vi "Treat Command.vi"(8 "error in (no error)":errorcluster, 11 "Channel in":refnum<class "Channel.lvclass">) -> (0 "error out":errorcluster, 3 "Channel out":refnum<class "Channel.lvclass">)   [LabVIEW 2018, in "Channel.lvclass"]
doc: "Treat the commando received from the control interface."
uses:
  Channel.lvclass
  Channel.lvclass/Channel.ctl
  State Machine/CCS_State Machine.lvclass
  Simulated_CCD_Camera/Simulated Camera.lvclass
  RxTx/CCS_RxTx.lvclass
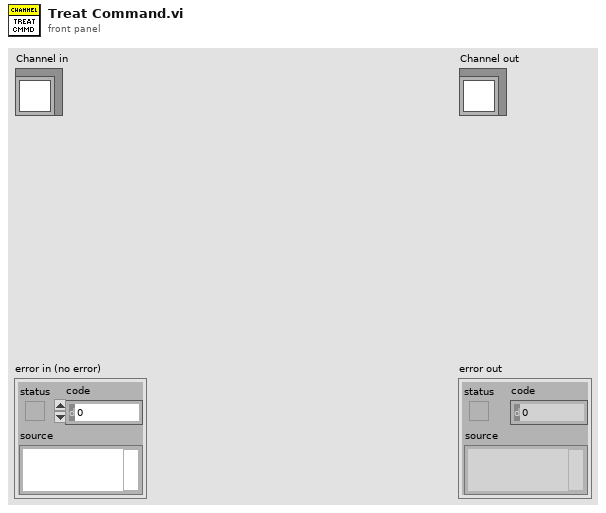
[diagram p1: front panel]
types:
  T1 = cluster{"CYCLES_DONE":u16, "LAST_IMAGE_NAME":string, "USED_DISK_SPACE":u16, "FRAMES_DONE":u16, "CCD_STATUS":string, "CURRENT_TEMPERATURE":i16, "TEMPERATURE_STATUS":string, "FRAME_EXPOSURE_TIME":sgl, "ERROR":bool, "SERIAL_NUMBER":u16, "ACQUIRING":bool, "IMAGE_INDEX":u32, "SEQS_DONE":u16}
  T2 = cluster{"COOLER_POWER_STATUS":u16, "TEMP":i32, "EXPTIME":dbl, "#FRAMES":u32, "#CYCLES":u32, "#SEQS":u32, "WAVEPLATE_POS":u16}
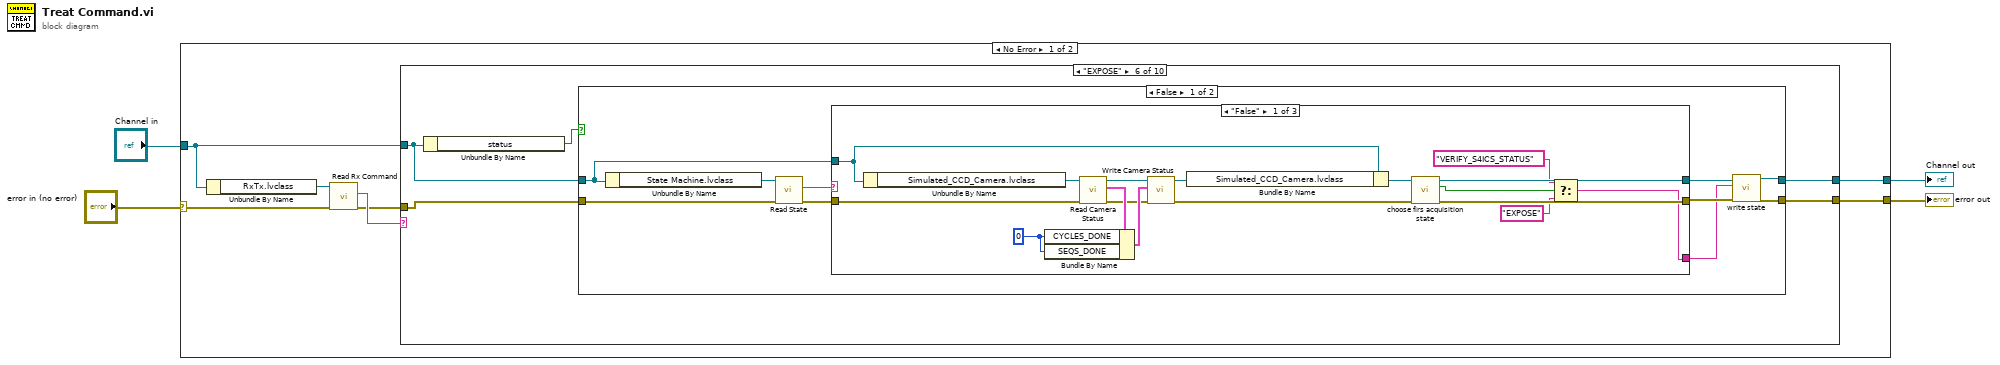
[diagram p0: block diagram]
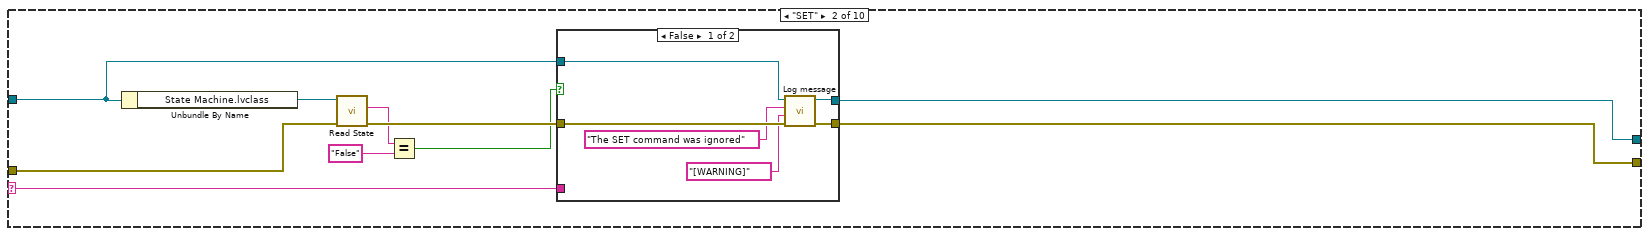
[diagram p3: hidden frame]
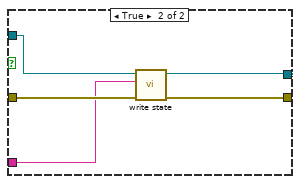
[diagram p4: hidden frame]
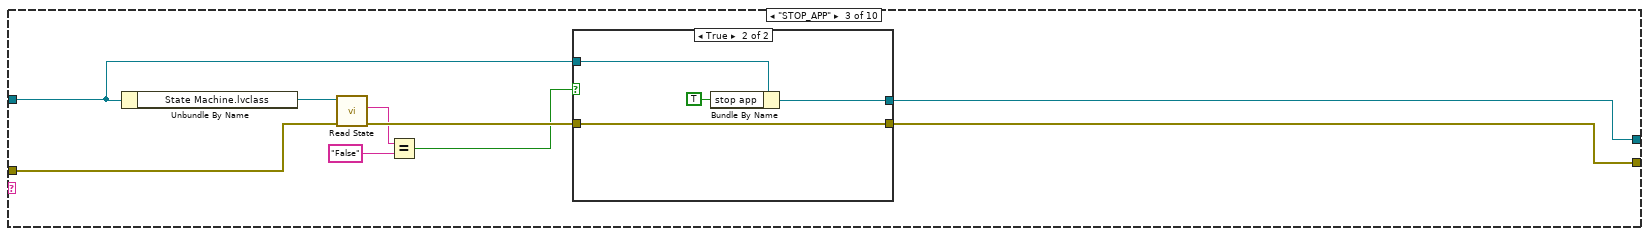
[diagram p5: hidden frame]
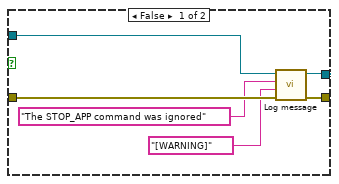
[diagram p6: hidden frame]
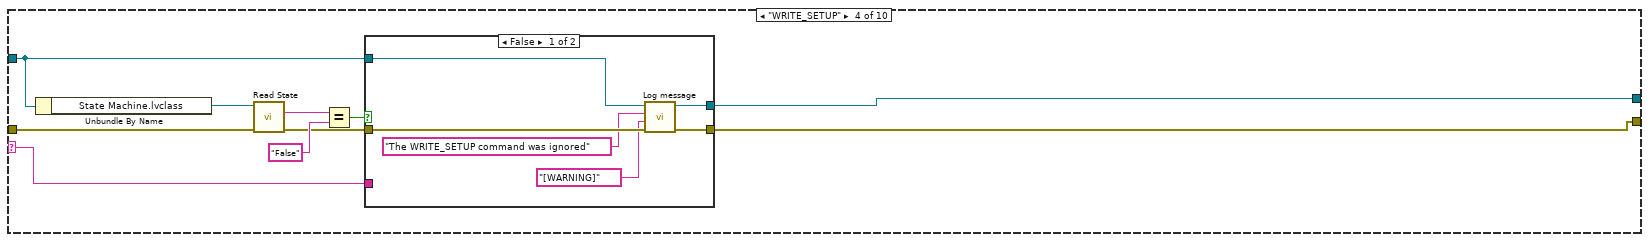
[diagram p7: hidden frame]
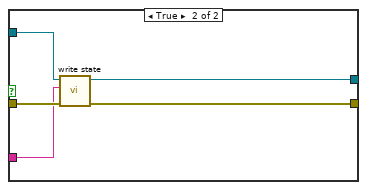
[diagram p8: hidden frame]
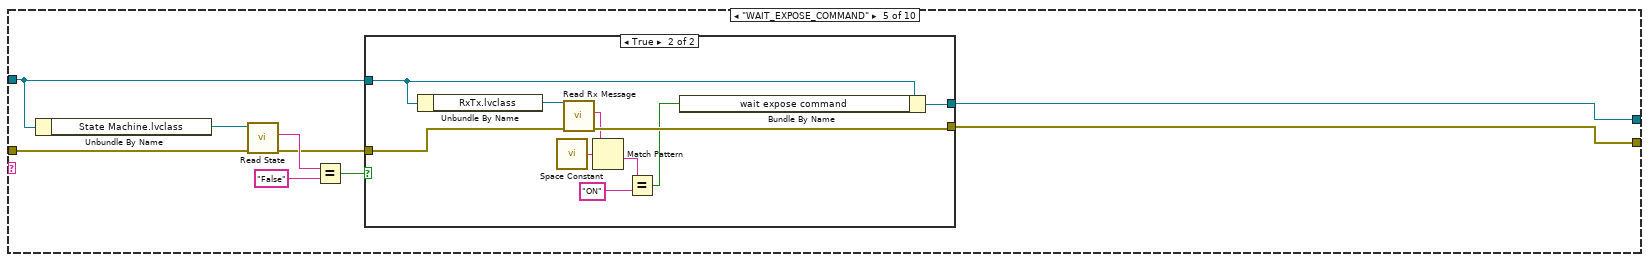
[diagram p9: hidden frame]
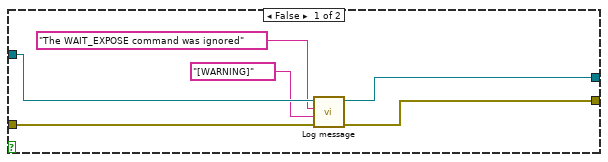
[diagram p10: hidden frame]
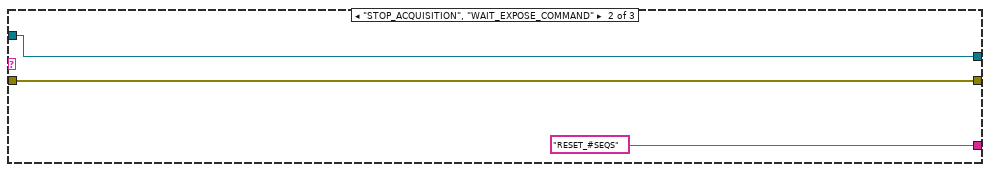
[diagram p11: hidden frame]
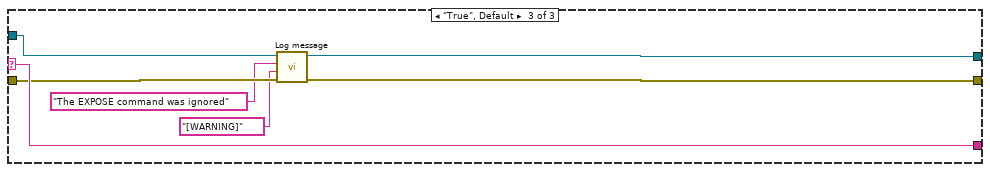
[diagram p12: hidden frame]
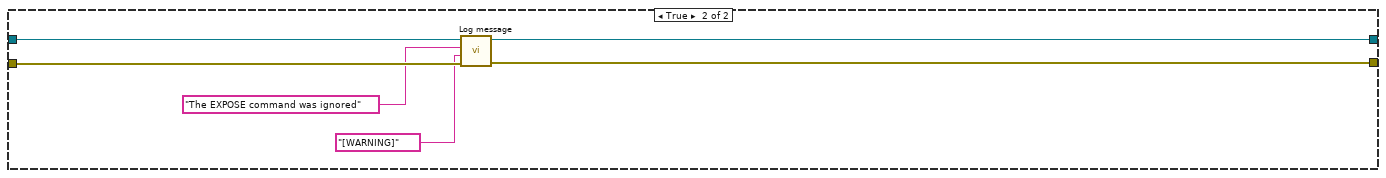
[diagram p13: hidden frame]
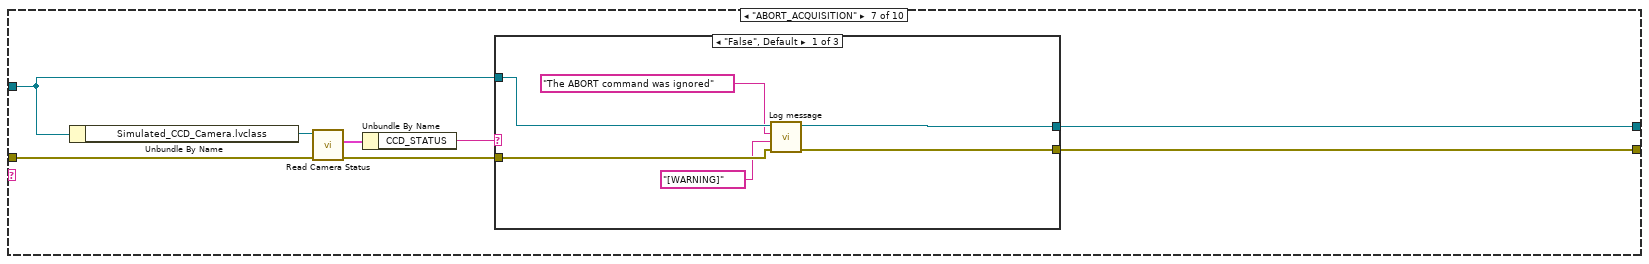
[diagram p14: hidden frame]
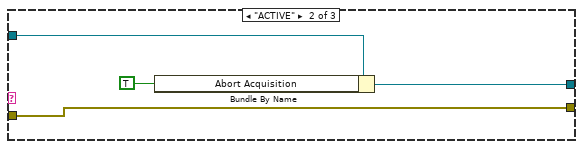
[diagram p15: hidden frame]
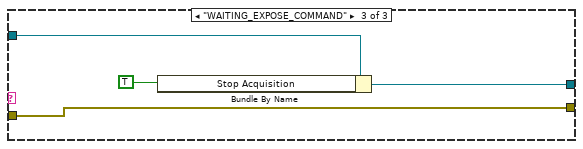
[diagram p16: hidden frame]
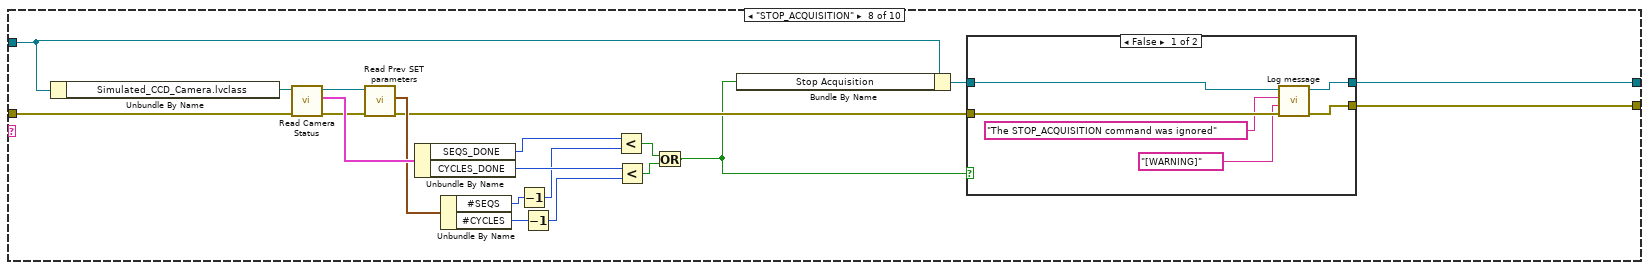
[diagram p17: hidden frame]
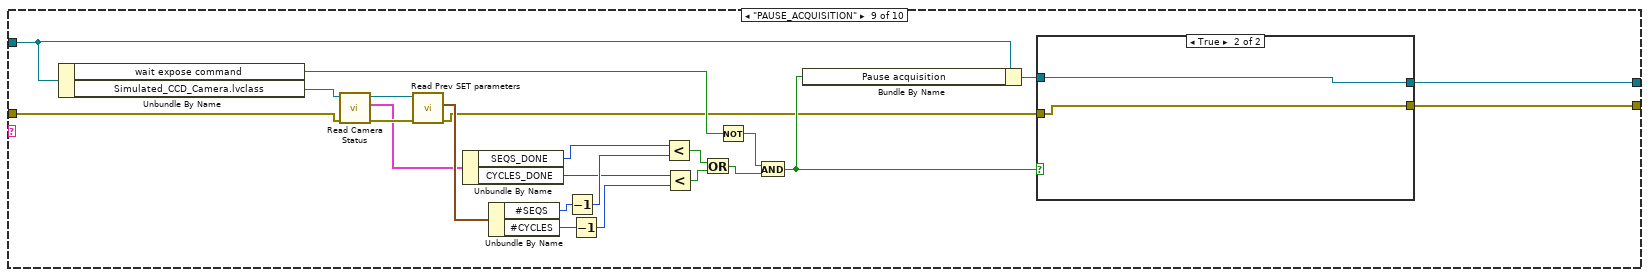
[diagram p19: hidden frame]
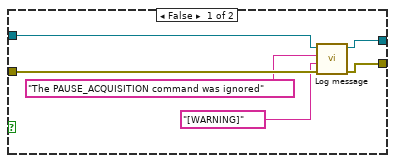
[diagram p20: hidden frame]
diagram:
  n1 = case shown="No Error" "error in (no error)" {
    selector: "error in (no error)" -> [w10 w248]
    tunnel: [w7 w248] -> w3
    tunnel: [w8 w247] -> w1
    tunnel: "Channel in" -> [w6 w247]
    frame No Error {
      n2 = Unbundle By Name(w6) -> ("RxTx.lvclass"=w11:refnum<class "CCS_RxTx.lvclass">)
      n3 = call "Read Rx Command.vi"("error in (no error)"=w10, "RxTx in"=w11) -> ("error out"=w5:errorcluster, "Rx Command"=w9:string)  [unwired: 7 in, 1 out]
      n4 = case shown="\"EXPOSE\"" w9 {
        selector: w9 -> [_ w15 _ w54 _ _ _ _ _ _]
        tunnel: w6 -> [w13 w17 w37 w58 w78 w101 w155 w189 w220 w238]
        tunnel: [w13 w19 w39 w57 w76 w103 w154 w179 w219 w236] -> w8
        tunnel: w5 -> [w12 w20 w40 w61 w81 w102 w152 w184 w199 w237]
        tunnel: [w12 w18 w38 w56 w75 w104 w148 w178 w218 w235] -> w7
        frame "False", Default {
        }
        frame "SET" {
          n5 = Unbundle By Name(w17) -> ("State Machine.lvclass"=w22:refnum<class "CCS_State Machine.lvclass">)
          n6 = call-dynamic "Read State.vi"("error in (no error)"=w20, "State Machine in"=w22) -> ("error out"=w23:errorcluster, "State"=w16:string)  [unwired: 7 in, 1 out]
          n7 = Equal?(x=w16, y="False") -> (x = y?=w14:bool)
          n8 = case shown="False" w14 {
            tunnel: w23 -> [w29 w31]
            tunnel: [w27 w33] -> w19
            tunnel: [w28 w32] -> w18
            tunnel: w17 -> [w26 w34]
            tunnel: w15 -> [_ w30]
            frame False {
              n9 = call "Log message.vi"("error in (no error)"=w29, "message type"="[WARNING]", "String"="The SET command was ignored", "Channel in"=w26) -> ("error out"=w28:errorcluster, "Channel out"=w27:refnum<class "Channel.lvclass">)  [unwired: 6 in]
            }
            frame True {
              n10 = call "write state.vi"("error in (no error)"=w31, "state"=w30, "Channel in"=w34) -> ("error out"=w32:errorcluster, "Channel out"=w33:refnum<class "Channel.lvclass">)  [unwired: 7 in]
            }
          }
        }
        frame "STOP_APP" {
          n11 = Unbundle By Name(w37) -> ("State Machine.lvclass"=w42:refnum<class "CCS_State Machine.lvclass">)
          n12 = call-dynamic "Read State.vi"("error in (no error)"=w40, "State Machine in"=w42) -> ("error out"=w43:errorcluster, "State"=w36:string)  [unwired: 7 in, 1 out]
          n13 = Equal?(x=w36, y="False") -> (x = y?=w35:bool)
          n14 = case shown="True" w35 {
            tunnel: w43 -> [w49 w53]
            tunnel: [w47 w51] -> w39
            tunnel: [w48 w53] -> w38
            tunnel: w37 -> [w46 w52]
            frame False {
              n15 = call "Log message.vi"("error in (no error)"=w49, "message type"="[WARNING]", "String"="The STOP_APP command was ignored", "Channel in"=w46) -> ("error out"=w48:errorcluster, "Channel out"=w47:refnum<class "Channel.lvclass">)  [unwired: 6 in]
            }
            frame True {
              n16 = Bundle By Name(cluster=w52, "stop app"=TRUE) -> (w51:refnum<class "Channel.lvclass">)
            }
          }
        }
        frame "WRITE_SETUP" {
          n17 = Unbundle By Name(w58) -> ("State Machine.lvclass"=w63:refnum<class "CCS_State Machine.lvclass">)
          n18 = call-dynamic "Read State.vi"("error in (no error)"=w61, "State Machine in"=w63) -> ("error out"=w59:errorcluster, "State"=w55:string)  [unwired: 7 in, 1 out]
          n19 = Equal?(x=w55, y="False") -> (x = y?=w60:bool)
          n20 = case shown="False" w60 {
            tunnel: w59 -> [w68 w74]
            tunnel: [w66 w72] -> w57
            tunnel: [w67 w73] -> w56
            tunnel: w58 -> [w69 w71]
            tunnel: w54 -> [_ w70]
            frame False {
              n21 = call "Log message.vi"("error in (no error)"=w68, "message type"="[WARNING]", "String"="The WRITE_SETUP command was ignored", "Channel in"=w69) -> ("error out"=w67:errorcluster, "Channel out"=w66:refnum<class "Channel.lvclass">)  [unwired: 6 in]
            }
            frame True {
              n22 = call "write state.vi"("error in (no error)"=w74, "state"=w70, "Channel in"=w71) -> ("error out"=w73:errorcluster, "Channel out"=w72:refnum<class "Channel.lvclass">)  [unwired: 7 in]
            }
          }
        }
        frame "WAIT_EXPOSE_COMMAND" {
          n23 = Unbundle By Name(w78) -> ("State Machine.lvclass"=w83:refnum<class "CCS_State Machine.lvclass">)
          n24 = call-dynamic "Read State.vi"("error in (no error)"=w81, "State Machine in"=w83) -> ("error out"=w77:errorcluster, "State"=w80:string)  [unwired: 7 in, 1 out]
          n25 = Equal?(x=w80, y="False") -> (x = y?=w79:bool)
          n26 = case shown="True" w79 {
            tunnel: w78 -> [w89 w98]
            tunnel: w77 -> [w86 w99]
            tunnel: [w88 w94] -> w76
            tunnel: [w87 w95] -> w75
            frame False {
              n27 = call "Log message.vi"("error in (no error)"=w86, "message type"="[WARNING]", "String"="The WAIT_EXPOSE command was ignored", "Channel in"=w89) -> ("error out"=w87:errorcluster, "Channel out"=w88:refnum<class "Channel.lvclass">)  [unwired: 6 in]
            }
            frame True {
              n28 = Unbundle By Name(w98) -> ("RxTx.lvclass"=w97:refnum<class "CCS_RxTx.lvclass">)
              n29 = call <vilib>:"Space Constant.vi"() -> ("String"=w90:string)
              n30 = call "Read Rx Message.vi"("error in (no error)"=w99, "RxTx in"=w97) -> ("error out"=w95:errorcluster, "Rx Message"=w92:string)  [unwired: 7 in, 1 out]
              n31 = Match Pattern(string=w92, regular expression=w90) -> (after substring=w91:string)  [unwired: 1 in, 3 out]
              n32 = Equal?(x=w91, y="ON") -> (x = y?=w93:bool)
              n33 = Bundle By Name(cluster=w98, "wait expose command"=w93) -> (w94:refnum<class "Channel.lvclass">)
            }
          }
        }
        frame "EXPOSE" {
          n34 = Unbundle By Name(w101) -> ("status"=w100:bool)
          n35 = case shown="False" w100 {
            tunnel: [w107 w144] -> w104
            tunnel: w102 -> [w113 w146]
            tunnel: w101 -> [w111 w147]
            tunnel: [w108 w145] -> w103
            frame False {
              n36 = Unbundle By Name(w111) -> ("State Machine.lvclass"=w114:refnum<class "CCS_State Machine.lvclass">)
              n37 = call-dynamic "Read State.vi"("error in (no error)"=w113, "State Machine in"=w114) -> ("error out"=w110:errorcluster, "State"=w112:string)  [unwired: 7 in, 1 out]
              n38 = case shown="\"False\"" w112 {
                selector: w112 -> [_ _ w141]
                tunnel: w111 -> [w124 w133 w140]
                tunnel: w110 -> [w125 w134 w137]
                tunnel: [w121 w133 w139] -> w109
                tunnel: [w120 w134 w138] -> w106
                tunnel: [w116 "RESET_#SEQS" w141] -> w105
                frame "False" {
                  w126 = u16 0 ("CUBES_DONE")
                  n39 = Unbundle By Name(w124) -> ("Simulated_CCD_Camera.lvclass"=w127:refnum<class "Simulated Camera.lvclass">)
                  n40 = call "Read Camera Status.vi"("error in (no error)"=w125, "CCDCamera in"=w127) -> ("error out"=w128:errorcluster, "Camera Status"=w130:T1, "CCDCamera out"=w131:refnum<class "Simulated Camera.lvclass">)  [unwired: 7 in]
                  n41 = Bundle By Name(cluster=w130, "CYCLES_DONE"=w126, "SEQS_DONE"=w126) -> (w129:T1)
                  n42 = call "Write Camera Status.vi"("error in (no error)"=w128, "Camera Status"=w129, "CCDCamera in"=w131) -> ("error out"=w119:errorcluster, "CCDCamera out"=w123:refnum<class "Simulated Camera.lvclass">)  [unwired: 7 in]
                  n43 = Bundle By Name(cluster=w124, "Simulated_CCD_Camera.lvclass"=w123) -> (w122:refnum<class "Channel.lvclass">)
                  n44 = call "choose firs acquisition state.vi"("error in (no error)"=w119, "Channel in"=w122) -> ("error out"=w120:errorcluster, "verify S4ICS status"=w115:bool, "Channel out"=w121:refnum<class "Channel.lvclass">)  [unwired: 7 in]
                  n45 = Select(t="VERIFY_S4ICS_STATUS" ("x"), s=w115, f="EXPOSE" ("x")) -> (s? t:f=w116:string)
                }
                frame "STOP_ACQUISITION", "WAIT_EXPOSE_COMMAND" {
                }
                frame "True", Default {
                  n46 = call "Log message.vi"("error in (no error)"=w137, "message type"="[WARNING]", "String"="The EXPOSE command was ignored", "Channel in"=w140) -> ("error out"=w138:errorcluster, "Channel out"=w139:refnum<class "Channel.lvclass">)  [unwired: 6 in]
                }
              }
              n47 = call "write state.vi"("error in (no error)"=w106, "state"=w105, "Channel in"=w109) -> ("error out"=w107:errorcluster, "Channel out"=w108:refnum<class "Channel.lvclass">)  [unwired: 7 in]
            }
            frame True {
              n48 = call "Log message.vi"("error in (no error)"=w146, "message type"="[WARNING]", "String"="The EXPOSE command was ignored" ("Message to log"), "Channel in"=w147) -> ("error out"=w144:errorcluster, "Channel out"=w145:refnum<class "Channel.lvclass">)  [unwired: 6 in]
            }
          }
        }
        frame "ABORT_ACQUISITION" {
          n49 = Unbundle By Name(w155) -> ("Simulated_CCD_Camera.lvclass"=w151:refnum<class "Simulated Camera.lvclass">)
          n50 = call "Read Camera Status.vi"("error in (no error)"=w152, "CCDCamera in"=w151) -> ("error out"=w149:errorcluster, "Camera Status"=w153:T1)  [unwired: 7 in, 1 out]
          n51 = Unbundle By Name(w153) -> ("CCD_STATUS"=w150:string)
          n52 = case shown="\"False\", Default" w150 {
            tunnel: w155 -> [w158 w165 w169]
            tunnel: [w159 w164 w168] -> w154
            tunnel: w149 -> [w161 w162 w166]
            tunnel: [w160 w162 w166] -> w148
            frame "False", Default {
              n53 = call "Log message.vi"("error in (no error)"=w161, "message type"="[WARNING]", "String"="The ABORT command was ignored" ("Message to log"), "Channel in"=w158) -> ("error out"=w160:errorcluster, "Channel out"=w159:refnum<class "Channel.lvclass">)  [unwired: 6 in]
            }
            frame "ACTIVE" {
              n54 = Bundle By Name(cluster=w165, "Abort Acquisition"=TRUE) -> (w164:refnum<class "Channel.lvclass">)
            }
            frame "WAITING_EXPOSE_COMMAND" {
              n55 = Bundle By Name(cluster=w169, "Stop Acquisition"=TRUE ("Abort Acquisition")) -> (w168:refnum<class "Channel.lvclass">)
            }
          }
        }
        frame "STOP_ACQUISITION" {
          n56 = Unbundle By Name(w189) -> ("Simulated_CCD_Camera.lvclass"=w185:refnum<class "Simulated Camera.lvclass">)
          n57 = call "Read Camera Status.vi"("error in (no error)"=w184, "CCDCamera in"=w185) -> ("error out"=w183:errorcluster, "Camera Status"=w188:T1, "CCDCamera out"=w182:refnum<class "Simulated Camera.lvclass">)  [unwired: 7 in]
          n58 = call-dynamic "Read Prev SET parameters.vi"("error in (no error)"=w183, "Simulated_CCD_Camera in"=w182) -> ("error out"=w180:errorcluster, "Prev SET parameters"=w186:T2)  [unwired: 7 in, 1 out]
          n59 = Unbundle By Name(w188) -> ("SEQS_DONE"=w174:u16, "CYCLES_DONE"=w187:u16)
          n60 = Unbundle By Name(w186) -> ("#SEQS"=w175:u32, "#CYCLES"=w177:u32)
          n61 = Decrement(x=w175) -> (x-1=w173:u32)
          n62 = Decrement(x=w177) -> (x-1=w176:u32)
          n63 = Less?(x=w174, y=w173) -> (x < y?=w171:bool)
          n64 = Less?(x=w187, y=w176) -> (x < y?=w172:bool)
          n65 = Or(x=w171, y=w172) -> (x .or. y?=w170:bool)
          n66 = Bundle By Name(cluster=w189, "Stop Acquisition"=w170) -> (w181:refnum<class "Channel.lvclass">)
          n67 = case shown="False" w170 {
            tunnel: w181 -> [w195 w197]
            tunnel: w180 -> [w194 w196]
            tunnel: [w192 w197] -> w179
            tunnel: [w193 w196] -> w178
            frame False {
              n68 = call "Log message.vi"("error in (no error)"=w194, "message type"="[WARNING]", "String"="The STOP_ACQUISITION command was ignored", "Channel in"=w195) -> ("error out"=w193:errorcluster, "Channel out"=w192:refnum<class "Channel.lvclass">)  [unwired: 6 in]
            }
            frame True {
            }
          }
        }
        frame "PAUSE_ACQUISITION" {
          n69 = Unbundle By Name(w220) -> ("wait expose command"=w215:bool, "Simulated_CCD_Camera.lvclass"=w200:refnum<class "Simulated Camera.lvclass">)
          n70 = call "Read Camera Status.vi"("error in (no error)"=w199, "CCDCamera in"=w200) -> ("error out"=w205:errorcluster, "Camera Status"=w202:T1, "CCDCamera out"=w206:refnum<class "Simulated Camera.lvclass">)  [unwired: 7 in]
          n71 = call-dynamic "Read Prev SET parameters.vi"("error in (no error)"=w205, "Simulated_CCD_Camera in"=w206) -> ("error out"=w198:errorcluster, "Prev SET parameters"=w204:T2)  [unwired: 7 in, 1 out]
          n72 = Unbundle By Name(w202) -> ("SEQS_DONE"=w210:u16, "CYCLES_DONE"=w203:u16)
          n73 = Unbundle By Name(w204) -> ("#SEQS"=w209:u32, "#CYCLES"=w207:u32)
          n74 = Decrement(x=w209) -> (x-1=w211:u32)
          n75 = Decrement(x=w207) -> (x-1=w208:u32)
          n76 = Less?(x=w210, y=w211) -> (x < y?=w213:bool)
          n77 = Less?(x=w203, y=w208) -> (x < y?=w212:bool)
          n78 = Or(x=w213, y=w212) -> (x .or. y?=w201:bool)
          n79 = Not(x=w215) -> (.not. x?=w216:bool)
          n80 = And(x=w216, y=w201) -> (x .and. y?=w214:bool)
          n81 = Bundle By Name(cluster=w220, "Pause acquisition"=w214) -> (w217:refnum<class "Channel.lvclass">)
          n82 = case shown="True" w214 {
            tunnel: w217 -> [w226 w228]
            tunnel: w198 -> [w225 w227]
            tunnel: [w223 w228] -> w219
            tunnel: [w224 w227] -> w218
            frame False {
              n83 = call "Log message.vi"("error in (no error)"=w225, "message type"="[WARNING]", "String"="The PAUSE_ACQUISITION command was ignored", "Channel in"=w226) -> ("error out"=w224:errorcluster, "Channel out"=w223:refnum<class "Channel.lvclass">)  [unwired: 6 in]
            }
            frame True {
            }
          }
        }
        frame "RESUME_ACQUISITION" {
          n84 = Unbundle By Name(w238) -> ("Pause acquisition"=w231:bool, "wait expose command"=w232:bool)
          n85 = Bundle By Name(cluster=w238, "Pause acquisition"=FALSE ("Acquisition control.Pause acquisition")) -> (w234:refnum<class "Channel.lvclass">)
          n86 = Not(x=w231) -> (.not. x?=w230:bool)
          n87 = Or(x=w230, y=w232) -> (x .or. y?=w229:bool)
          n88 = case shown="False" w229 {
            tunnel: w234 -> [w240 w246]
            tunnel: w237 -> [w239 w245]
            tunnel: [w240 w243] -> w236
            tunnel: [w239 w244] -> w235
            frame False {
            }
            frame True {
              n89 = call "Log message.vi"("error in (no error)"=w245, "message type"="[WARNING]", "String"="The RESUME_ACQUISITION command was ignored", "Channel in"=w246) -> ("error out"=w244:errorcluster, "Channel out"=w243:refnum<class "Channel.lvclass">)  [unwired: 6 in]
            }
          }
        }
      }
    }
    frame Error {
    }
  }
  "error out" <- w3
  "Channel out" <- w1
